vi "Draw_Bars.vi"(6 "3D?":bool=TRUE, 7 "White Plot":dbl[][](array[numeric]), 8 "reference":refnum<vi>, 9 "Top grid":cluster{"x":dbl, "y":dbl}[][](array[cluster]), 10 "Bottom grid":cluster{"x":dbl, "y":dbl}[][](array[cluster]), 11 "picture in":picture) -> (3 "picture out":picture)   [LabVIEW 2022 SP3]
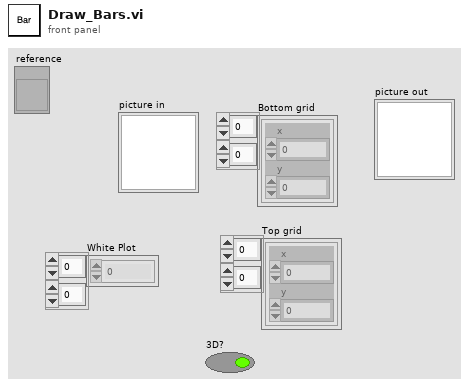
[diagram p1: front panel]
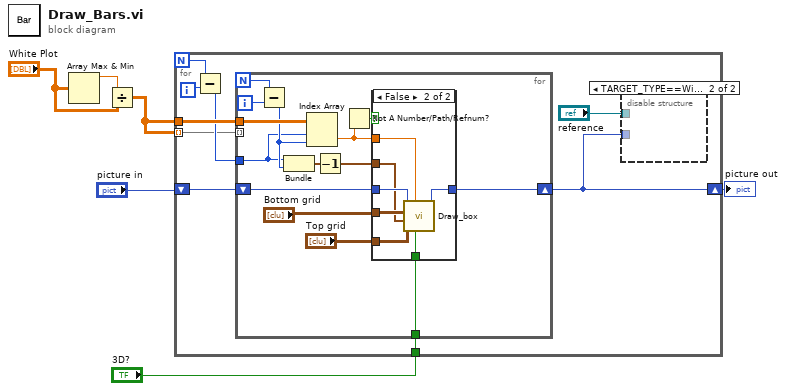
[diagram p0: block diagram]
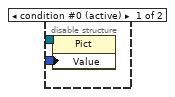
[diagram p2: hidden frame]
diagram:
  n1 = Array Max & Min(array="White Plot") -> (max value=w2:dbl)  [unwired: 3 out]
  n2 = Divide(x="White Plot", y=w2) -> (x/y=w4:dbl[][])
  n3 = for {
    N -> [w13]
    shift-right: [w7] -> w3
    shift-left: "picture in" -> [w15]
    tunnel: w4 -> [w14]
    tunnel: w4 -> [w10] mode=indexing
    tunnel: "3D?" -> [w9]
    i -> [w12]
    n4 = Subtract(x=w13, y=w12) -> (x-y=w11:i32)
    n5 = for {
      N -> [w29]
      shift-right: [w18] -> w7
      shift-left: w15 -> [w31]
      tunnel: w14 -> [w26]
      tunnel: w11 -> [w24]
      tunnel: w10 -> [_] mode=indexing
      tunnel: w9 -> [w19]
      i -> [w28]
      n6 = Subtract(x=w29, y=w28) -> (x-y=w25:i32)
      n7 = Bundle(w24, w25) -> (w30:cluster{i32, i32})  [unwired: 1 in]
      n8 = Index Array(array=w26, index (row)=w24, index (col)=w25) -> (element=w22:dbl)
      n9 = Decrement(x=w30) -> (x-1=w27:cluster{i32, i32})
      n10 = Not A Number/Path/Refnum?(number/path/refnum=w22) -> (NaN/Path/Refnum?=w23:bool)
      n11 = case shown="False" w23 {
        tunnel: "Bottom grid" -> [_ w39]
        tunnel: w31 -> [w32 w38]
        tunnel: "Top grid" -> [_ w37]
        tunnel: [w32 w36] -> w18
        tunnel: w27 -> [_ w35]
        tunnel: w22 -> [_ w34]
        tunnel: w19 -> [_ w33]
        frame True {
        }
        frame False {
          n12 = call "Draw_box.vi"("Z Value"=w34, "3D?"=w33, "Top"=w37, "element"=w35, "Base"=w39, "picture in"=w38) -> ("picture out"=w36:picture)  [unwired: 4 in, 1 out]
        }
      }
    }
    n13 = disable-structure shown="TARGET_TYPE==Windows" {
      disable-tunnel: "reference" -> [w17 _]
      disable-tunnel: w7 -> [w16 _]
      frame condition #0 (active) {
        n14 = property class="Pict"(reference=w17, "Value"=w16) -> ()  [unwired: 1 in, 2 out]
      }
      frame condition #1 {
      }
    }
  }
  "picture out" <- w3
